vi "NanotecSMCPD.contents.vi"() -> ()   [LabVIEW 2014, in "NanotecSMCPD.lvlib"]
doc: "Contains \"all\" VIs- needed for building an application"
uses:
  NanotecSMCPD.lvlib
panel:
  out "error out":errorcluster
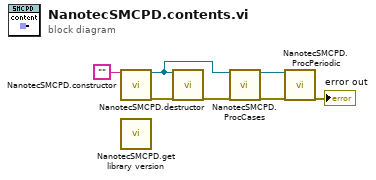
[diagram p0: block diagram]
diagram:
  n1 = call "NanotecSMCPD.constructor.vi"("name"="") -> ("i ref out"=w3:refnum<vi>, "error out"=w7:errorcluster)  [unwired: 16 in, 1 out]
  n2 = call "NanotecSMCPD.get library version.vi"() -> ()  [unwired: 1 in, 1 out]
  n3 = call "NanotecSMCPD.destructor.vi"("i ref in"=w3, "error in (no error)"=w7) -> ("error out"=w6:errorcluster)  [unwired: 17 in]
  n4 = call "NanotecSMCPD.ProcCases.vi"("i ref in"=w3, "error in (no error)"=w6) -> ("i ref out"=w4:refnum<vi>, "error out"=w5:errorcluster)  [unwired: 15 in, 1 out]
  n5 = call "NanotecSMCPD.ProcPeriodic.vi"("i ref in"=w4, "error in (no error)"=w5) -> ("error out"=→"error out":errorcluster)  [unwired: 15 in, 2 out]
